vi "GetGlobalVIPathFromURL.vi"(10 "diagram":refnum<vi>, 11 "URL":string) -> (3 "path":path)   [LabVIEW 2020]
uses:
  <vilib>/variable/NI_Variable.lvlib
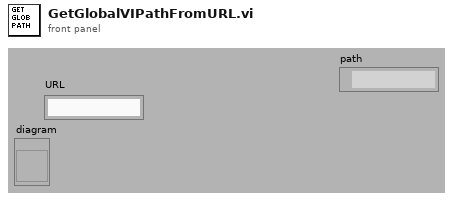
[diagram p1: front panel]
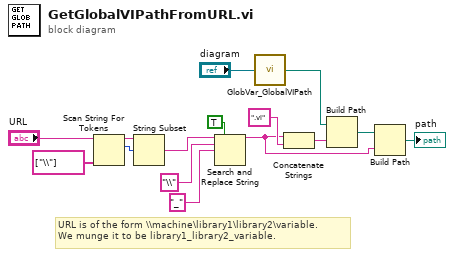
[diagram p0: block diagram]
diagram:
  # "URL is of the form \\\\machine\\library1\\library2\\variable.\nWe munge it to be library1_library2_variable."
  n1 = Scan String For Tokens(6:string[] ["\\"] ("delimiters (\\s,\\t,\\r,\\n)"), 9:"URL") -> (2:w8:i32, 3:w7:string)  [unwired: 4 in, 2 out]
  n2 = String Subset(string=w7, offset (0)=w8) -> (substring=w9:string)  [unwired: 1 in]
  n3 = Search and Replace String(replace all?=TRUE ("replace all? (Yes)"), input string=w9, search string="\\", replace string="_" ("replace string (\"\")")) -> (result string=w5:string)  [unwired: 4 in, 3 out]
  n4 = call <vilib>:"GlobVar_GlobalVIPath.vi"("diagram"="diagram") -> ("path"=w3:path)
  n5 = Concatenate Strings(w5, ".vi" ("string")) -> (w14:string)
  n6 = Build Path(base path=w3, name or relative path=w14) -> (appended path=w15:path)
  n7 = Build Path(base path=w15, name or relative path=w5) -> (appended path=→"path":path)
